vi "Database.Handler.ReconnectOne.vi"(8 "error in (no error)":errorcluster, 10 "Idx":i32, 11 "Data in":T1) -> (0 "error out":errorcluster, 3 "Data out":T1)   [LabVIEW 2016]
uses:
  Database.Handler.Data.ctl
  Database.Handler.Data.Status.ctl
  Database.Handler.Data.Sets.ctl
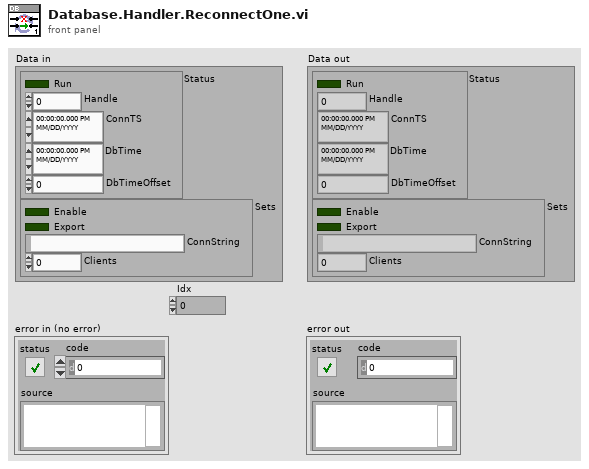
[diagram p1: front panel]
types:
  T1 = typedef "Database.Handler.Data.ctl" = cluster{"Status":T2, "Sets":T3}
  T2 = typedef "Database.Handler.Data.Status.ctl" = cluster{"Run":bool, "Handle":i32, "ConnTS":timestamp, "DbTime":timestamp, "DbTimeOffset":dbl}
  T3 = typedef "Database.Handler.Data.Sets.ctl" = cluster{"Enable":bool, "Export":bool, "ConnString":string, "Clients":i32}
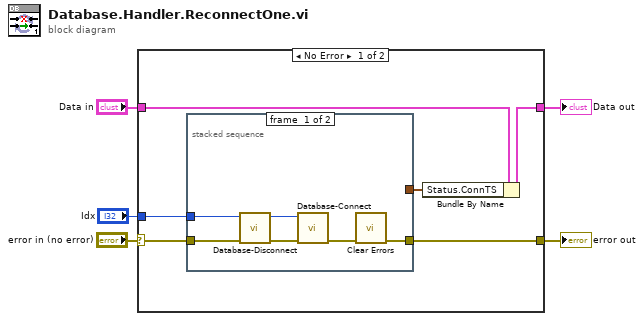
[diagram p0: block diagram]
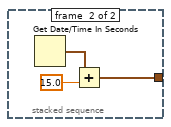
[diagram p2: hidden frame]
diagram:
  n1 = case shown="No Error" "error in (no error)" {
    selector: "error in (no error)" -> [w11 w21]
    tunnel: [w8 w20] -> w5
    tunnel: "Data in" -> [w9 w20]
    tunnel: [w7 w21] -> w3
    tunnel: "Idx" -> [w6 _]
    frame No Error {
      n2 = stacked-sequence {
        tunnel: w11 -> [w16 _]
        tunnel: [w12 _] -> w7
        tunnel: w6 -> [w13 _]
        tunnel: [_ w17] -> w10
        frame #0 {
          n3 = call "Database-Disconnect.vi"("error in"=w16, "Idx"=w13) -> ("error out"=w15:errorcluster)  [unwired: 9 in]
          n4 = call "Database-Connect.vi"("error in"=w15, "Idx"=w13) -> ("error out"=w14:errorcluster)  [unwired: 9 in]
          n5 = call <vilib>:"Clear Errors.vi"("error in (no error)"=w14) -> ("error out"=w12:errorcluster)  [unwired: 5 in, 1 out]
        }
        frame #1 {
          n6 = Get Date/Time In Seconds() -> (seconds since 1Jan1904=w19:timestamp)
          n7 = Add(x=w19, y=15.0) -> (x+y=w17:timestamp)
        }
      }
      n8 = Bundle By Name(cluster=w9, "Status.ConnTS"=w10) -> (w8:T1)
    }
    frame Error {
    }
  }
  "Data out" <- w5
  "error out" <- w3
